vi "5492_YawParser.vi"(11 "Yaw":dbl) -> (3 "Parsed Yaw":dbl)   [LabVIEW 2016]
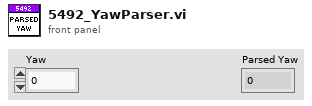
[diagram p1: front panel]
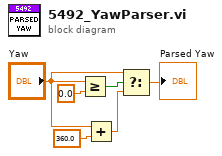
[diagram p0: block diagram]
diagram:
  n1 = Greater Or Equal?(x="Yaw", y=0.0) -> (x >= y?=w5:bool)
  n2 = Add(x="Yaw", y=360.0) -> (x+y=w1:dbl)
  n3 = Select(t="Yaw", s=w5, f=w1) -> (s? t:f=→"Parsed Yaw":dbl)
